vi "Get Cursor X positions.vi"(8 "error in":errorcluster, 11 "Timeline Graph":T1) -> (0 "error out":errorcluster, 1 "Right cursor pos.":dbl, 2 "Left cursor pos.":dbl, 3 "Timeline Graph out":T1, 4 "Cursors":cluster{"Left":dbl, "Right":dbl, "Span":dbl})   [LabVIEW 2017, in "XGrapher.xctl"]
doc: "Gets the x positions of the right and left cursors of the timeline graph"
uses:
  XGrapher.xctl
  Typedefs/Xctrl-Timeline graph ref.ctl
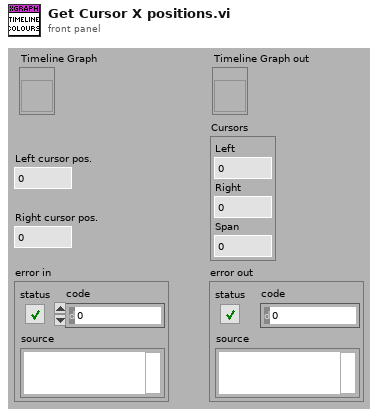
[diagram p1: front panel]
types:
  T1 = typedef "XGrapher.xctl/Xctrl-Timeline graph ref.ctl" = refnum<vi>
  T2 = cluster{"left":i16, "top":i16, "right":i16, "bottom":i16}
  T3 = cluster{"Cursor.Cursor X":dbl, "Cursor.Cursor X":dbl}
  T4 = cluster{"XScale.Maximum":dbl, "XScale.Maximum":dbl}
  T5 = cluster{"XScale.Minimum":dbl, "XScale.Minimum":dbl}
  T6 = cluster{"Cursor.Cursor X":dbl, "Cursor.Cursor X":dbl, dbl}
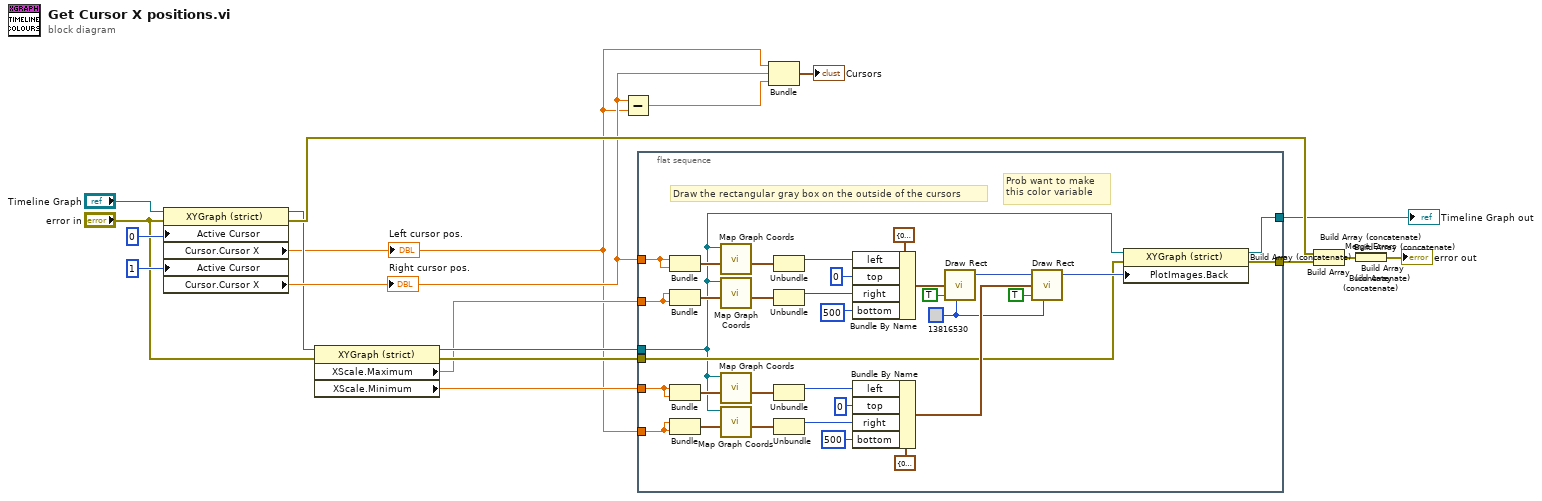
[diagram p0: block diagram]
diagram:
  n1 = property on="Property Node" class="XYGraph (strict)"(reference="Timeline Graph", error in="error in", "Active Cursor"=u32 0, "Active Cursor"=u32 1) -> (reference out=w6:T1, error out=w21:errorcluster, "Cursor.Cursor X"=w1:dbl, "Cursor.Cursor X"=w18:dbl)
  "Left cursor pos." <- w1
  "Right cursor pos." <- w18
  n2 = property on="Property Node" class="XYGraph (strict)"(reference=w6, error in="error in") -> (reference out=w5:T1, error out=w4:errorcluster, "XScale.Maximum"=w3:dbl, "XScale.Minimum"=w2:dbl)
  n3 = Subtract(x=w18, y=w1) -> (x-y=w17:dbl)
  n4 = flat-sequence {
    tunnel: w3 -> [w54]
    tunnel: w2 -> [w45]
    tunnel: w18 -> [w32]
    tunnel: w1 -> [w31]
    tunnel: w4 -> [w30]
    tunnel: [w29] -> w20
    tunnel: w5 -> [w26]
    tunnel: [w27] -> w9
    frame #0 {
      w28 = u32 13816530
      # "Prob want to make \nthis color variable"
      # "Draw the rectangular gray box on the outside of the cursors"
      n5 = Bundle("Cursor.Cursor X"=w32, "Cursor.Cursor X"=w32) -> (w43:T3)  [unwired: 1 in]
      n6 = Bundle("XScale.Maximum"=w54, "XScale.Maximum"=w54) -> (w38:T4)  [unwired: 1 in]
      n7 = Bundle("XScale.Minimum"=w45, "XScale.Minimum"=w45) -> (w51:T5)  [unwired: 1 in]
      n8 = Bundle("Cursor.Cursor X"=w31, "Cursor.Cursor X"=w31) -> (w48:T3)  [unwired: 1 in]
      n9 = call "Map Graph Coords.vi"("XY"=w43, "Timeline Graph in"=w26) -> ("Coords"=w42:cluster{i32, i32})  [unwired: 8 in, 1 out]
      n10 = call "Map Graph Coords.vi"("XY"=w38, "Timeline Graph in"=w26) -> ("Coords"=w39:cluster{i32, i32})  [unwired: 8 in, 1 out]
      n11 = call "Map Graph Coords.vi"("XY"=w51, "Timeline Graph in"=w26) -> ("Coords"=w52:cluster{i32, i32})  [unwired: 8 in, 1 out]
      n12 = call "Map Graph Coords.vi"("XY"=w48, "Timeline Graph in"=w26) -> ("Coords"=w49:cluster{i32, i32})  [unwired: 8 in, 1 out]
      n13 = Unbundle(w42) -> (w41:i32)  [unwired: 1 out]
      n14 = Unbundle(w39) -> (w37:i32)  [unwired: 1 out]
      n15 = Unbundle(w52) -> (w53:i32)  [unwired: 1 out]
      n16 = Unbundle(w49) -> (w50:i32)  [unwired: 1 out]
      n17 = Bundle By Name(cluster=T2 {"left"=0, "top"=0, "right"=0, "bottom"=0} ("rect"), "left"=w41, "top"=i16 0 ("left"), "right"=w37, "bottom"=i16 500) -> (w55:T2)
      n18 = Bundle By Name(cluster=T2 {"left"=0, "top"=0, "right"=0, "bottom"=0} ("rect"), "left"=w53, "top"=i16 0 ("left"), "right"=w50, "bottom"=i16 500) -> (w33:T2)
      n19 = call <vilib>:"Draw Rect.vi"("rect"=w55, "fill?(F)"=TRUE, "color(black)"=w28) -> ("new picture"=w35:picture)  [unwired: 6 in]
      n20 = call <vilib>:"Draw Rect.vi"("picture"=w35, "rect"=w33, "fill?(F)"=TRUE, "color(black)"=w28) -> ("new picture"=w34:picture)  [unwired: 5 in]
      n21 = property on="Property Node" class="XYGraph (strict)"(reference=w26, error in=w30, "PlotImages.Back"=w34) -> (reference out=w27:T1, error out=w29:errorcluster)
    }
  }
  n22 = Bundle("Cursor.Cursor X"=w1, "Cursor.Cursor X"=w18, w17) -> (→"Cursors":T6)  [unwired: 1 in]
  n23 = Build Array(w21, w20) -> (w16:errorcluster[])
  n24 = Build Array (concatenate)(w16) -> (w15:errorcluster[])
  n25 = Build Array (concatenate)(w15) -> (w14:errorcluster[])
  n26 = Build Array (concatenate)(w14) -> (w13:errorcluster[])
  n27 = Build Array (concatenate)(w13) -> (w12:errorcluster[])
  n28 = Build Array (concatenate)(w12) -> (w11:errorcluster[])
  n29 = Merge Errors(w11) -> (→"error out":errorcluster)
  "Timeline Graph out" <- w9
